vi "GigEIssueActionCommand.vi"(0 "pBroadcastAddress":i8[](array[numeric]), 5 "pstActionCmdInfo":T3, 11 "error in (no error)":errorcluster caption="错误输入（无错误）") -> (4 "function return":i32, 6 "nNumResults":u32, 8 "ActionCmdResultArray":T2(array[cluster]), 15 "error out":errorcluster caption="错误输出")   [LabVIEW 2013, in "MvCameraControl.lvlib"]
uses:
  MvCameraControl.lvlib
  MvCameraPatch.dll
panel:
  in  "ActionCmdResults":T1
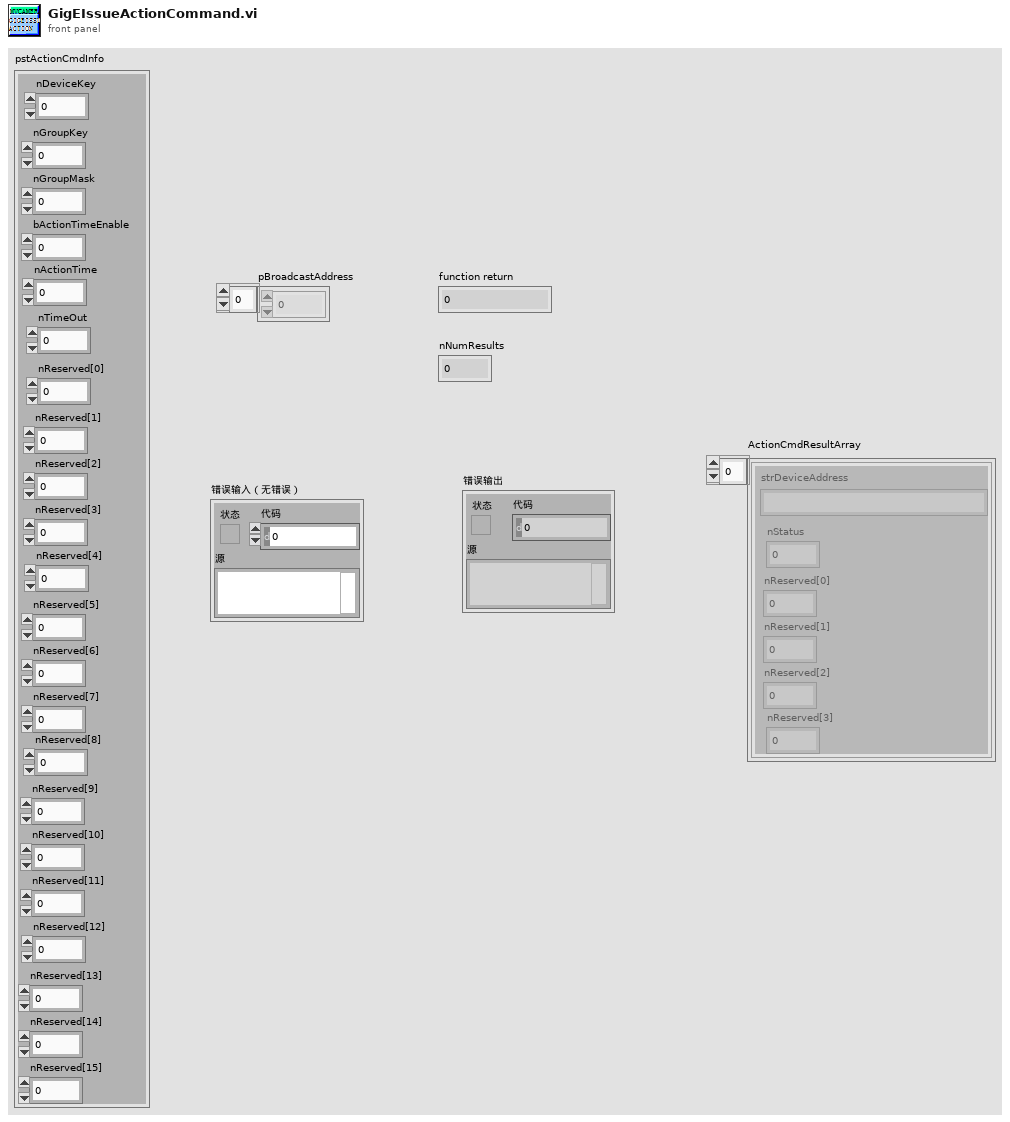
[diagram p1: front panel]
types:
  T1 = cluster{"strDeviceAddress":string, "nStatus":i32, "nReserved[0]":u32, "nReserved[1]":u32, "nReserved[2]":u32, "nReserved[3]":u32}
  T2 = cluster{"strDeviceAddress":string, "nStatus":i32, "nReserved[0]":u32, "nReserved[1]":u32, "nReserved[2]":u32, "nReserved[3]":u32}[]
  T3 = cluster{"nDeviceKey":u32, "nGroupKey":u32, "nGroupMask":u32, "bActionTimeEnable":u32, "nActionTime":i64, "nTimeOut":u32, "nReserved[3]":u32, "nReserved[2]":u32, "nReserved[1]":u32, "nReserved[0]":u32, "nReserved[7]":u32, "nReserved[6]":u32, "nReserved[5]":u32, "nReserved[4]":u32, "nReserved[11]":u32, "nReserved[10]":u32, "nReserved[9]":u32, "nReserved[8]":u32, "nReserved[15]":u32, "nReserved[14]":u32, "nReserved[13]":u32, "nReserved[12]":u32}
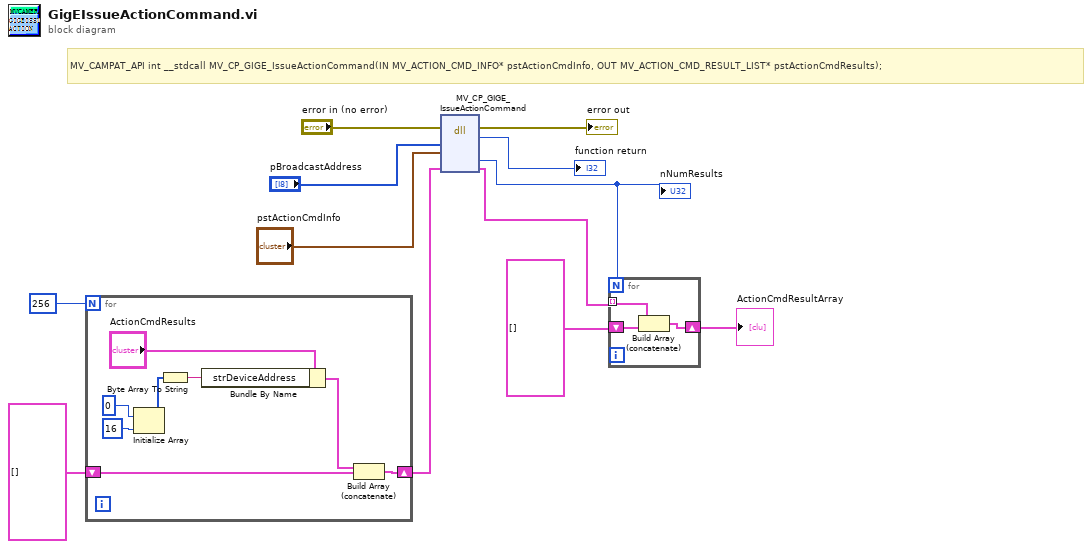
[diagram p0: block diagram]
diagram:
  # "MV_CAMPAT_API int __stdcall MV_CP_GIGE_IssueActionCommand(IN MV_ACTION_CMD_INFO* pstActionCmdInfo, OUT MV_ACTION_CMD_RESULT_LIST* pstActionCmdResults);"
  n1 = for {
    N: 256 -> [_]
    shift-right: [w13] -> w3
    shift-left: T2 [] -> [w14]
    n2 = Initialize Array(u8 0 ("元素"), 16 ("维数大小")) -> (w17:u8[])
    n3 = Byte Array To String(unsigned byte array=w17) -> (string=w16:string)
    n4 = Bundle By Name(cluster="ActionCmdResults", "strDeviceAddress"=w16) -> (w15:T1)
    n5 = Build Array (concatenate)(w15, w14) -> (w13:T2)
  }
  n6 = dll-call lib="MvCameraPatch.dll" fn="MV_CP_GIGE_IssueActionCommand"(error in="error in (no error)", "pBroadcastAddress"="pBroadcastAddress", "pstActionCmdInfo"="pstActionCmdInfo", "pActionCmdResultArray"=w3) -> (error out=→"error out":errorcluster, "返回类型"=→"function return":i32, "nNumResults"=w1:u32, "pActionCmdResultArray"=w2:T2)  [unwired: 5 in, 1 out]
  "nNumResults" <- w1
  n7 = for {
    N: w1 -> [_]
    shift-right: [w22] -> w4
    shift-left: T2 [] -> [w23]
    tunnel: w2 -> [w21] mode=indexing
    n8 = Build Array (concatenate)(w21, w23) -> (w22:T2)
  }
  "ActionCmdResultArray" <- w4
